vi "insert_data_in_Label_str.vi"(1 "dataToInsert":string, 2 "Input string":string, 3 "label name":string) -> (0 "Appended string":string)   [LabVIEW 2022 SP3]
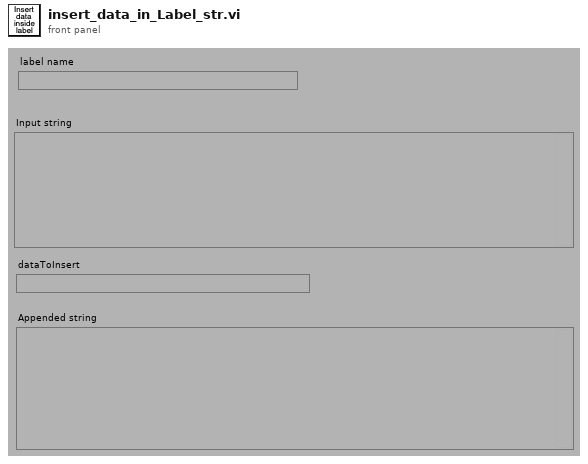
[diagram p1: front panel]
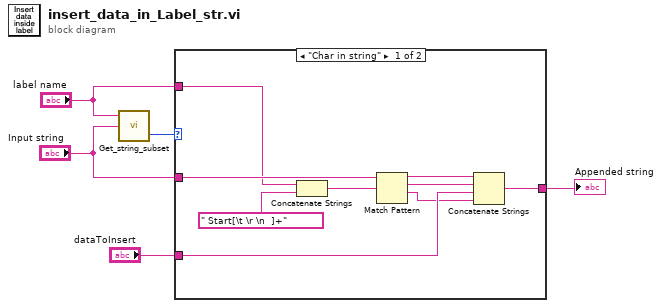
[diagram p0: block diagram]
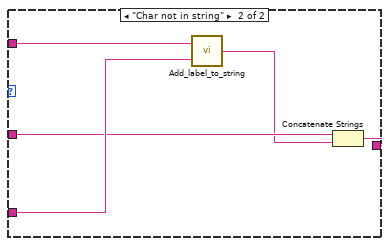
[diagram p2: hidden frame]
diagram:
  n1 = call "Get_string_subset.vi"("String to split"="Input string", "File Label"="label name") -> ("Status"=w1:enum16{"Char in string", "Char not in string"})  [unwired: 2 in, 1 out]
  n2 = case shown="\"Char in string\"" w1 {
    tunnel: "label name" -> [w12 w19]
    tunnel: "dataToInsert" -> [w11 w18]
    tunnel: [w13 w17] -> w4
    tunnel: "Input string" -> [w14 w16]
    frame "Char in string" {
      n3 = Concatenate Strings(w12, " Start[\t \r \n  ]+") -> (w9:string)
      n4 = Match Pattern(string=w14, regular expression=w9) -> (before substring=w8:string, match substring=w6:string, after substring=w7:string)  [unwired: 2 out]
      n5 = Concatenate Strings(w8, w6, w11, w7) -> (w13:string)
    }
    frame "Char not in string" {
      n6 = call "Add_label_to_string.vi"("String to write"=w18, "File Label"=w19) -> ("Output string"=w15:string)
      n7 = Concatenate Strings(w16, w15) -> (w17:string)
    }
  }
  "Appended string" <- w4
